vi "DAC Stop.vi"(8 "error in (no error)":errorcluster, 11 "DAC Inverter in":refnum<class "DAC Inverter.lvclass">) -> (0 "error out":errorcluster, 3 "DAC Inverter out":refnum<class "DAC Inverter.lvclass">)   [LabVIEW 2019, in "DAC.lvlib" / "DAC Inverter.lvclass"]
uses:
  DAC Inverter.lvclass
  DAC.lvclass
  <vilib>/NI/Modbus Library/API/Master/Modbus Master.lvclass
  C:/Users/wg/Documents/LV_Projects/test-stand/App/DAC/DAC.lvclass
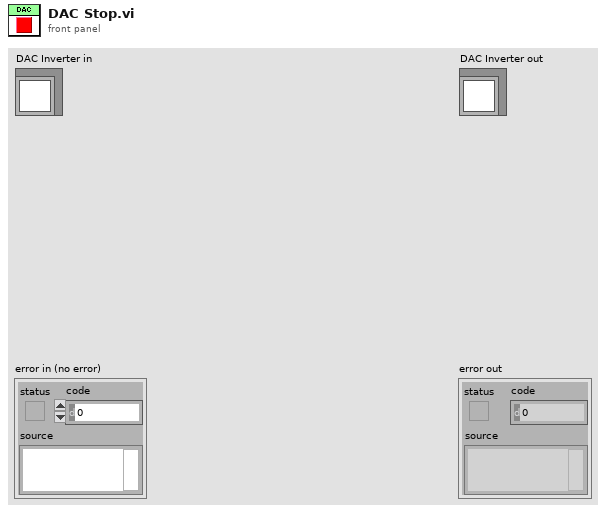
[diagram p1: front panel]
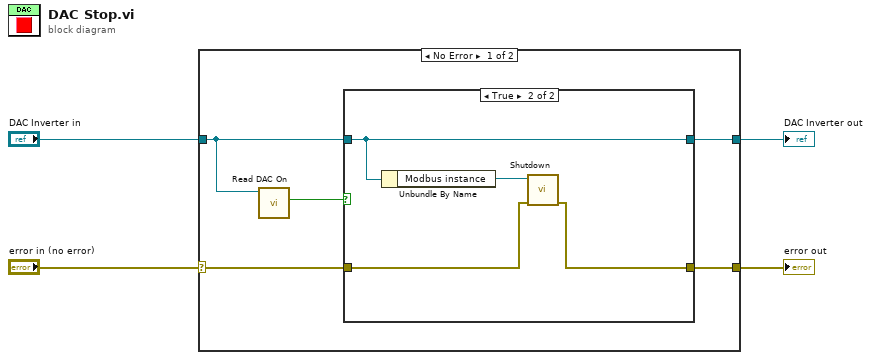
[diagram p0: block diagram]
diagram:
  n1 = case shown="No Error" "error in (no error)" {
    selector: "error in (no error)" -> [w6 w17]
    tunnel: [w5 w17] -> w1
    tunnel: [w7 w16] -> w3
    tunnel: "DAC Inverter in" -> [w9 w16]
    frame No Error {
      n2 = call "Read DAC On.vi"("DAC in"=w9) -> ("DAC On"=w8:bool)  [unwired: 8 in, 2 out]
      n3 = case shown="True" w8 {
        tunnel: w9 -> [w11 w15]
        tunnel: [w11 w15] -> w7
        tunnel: w6 -> [w10 w13]
        tunnel: [w10 w12] -> w5
        frame False {
        }
        frame True {
          n4 = Unbundle By Name(w15) -> ("Modbus instance"=w14:refnum<class "Modbus Master.lvclass">)
          n5 = call-dynamic "Shutdown.vi"("error in"=w13, "Modbus master in"=w14) -> ("error out"=w12:errorcluster)  [unwired: 9 in]
        }
      }
    }
    frame Error {
    }
  }
  "error out" <- w1
  "DAC Inverter out" <- w3
